vi "Example 3.vi"(8 "error in (no error)":errorcluster, 9 "export file path":path, 10 "target in":refnum<k24>, 11 "configuration file path":path) -> (0 "error out":errorcluster)   [LabVIEW 2018]
uses:
  NationalInstruments.VeriStand.SystemDefinitionAPI
  <vilib>/addons/VeriStand Custom Device Scripting APIs/Instrument Addon/API/TypeDefs/Message Settings.ctl
  <vilib>/addons/VeriStand Custom Device Scripting APIs/Instrument Addon/API/TypeDefs/Protection Types.ctl
  <vilib>/addons/VeriStand Custom Device Scripting APIs/Instrument Addon/API/TypeDefs/Single Channel Format Settings.ctl
  <vilib>/addons/VeriStand Custom Device Scripting APIs/Instrument Addon/API/TypeDefs/Command Settings.ctl
  <vilib>/NI Veristand/Custom Device API/Custom Device Item Ref.ctl
  <vilib>/addons/VeriStand Custom Device Scripting APIs/Instrument Addon/API/TypeDefs/Padding.ctl
  <vilib>/addons/VeriStand Custom Device Scripting APIs/Instrument Addon/API/TypeDefs/Array Type Cast Settings.ctl
  <vilib>/addons/VeriStand Custom Device Scripting APIs/Instrument Addon/API/TypeDefs/Array Element.ctl
  <vilib>/addons/VeriStand Custom Device Scripting APIs/Instrument Addon/Shared Directory/Type Cast Type.ctl
  <vilib>/addons/VeriStand Custom Device Scripting APIs/Instrument Addon/Shared Directory/Endian.ctl
  <vilib>/addons/VeriStand Custom Device Scripting APIs/Instrument Addon/API/Channels/Create Global MetaData Channel - Array - Type Cast.vi
  <vilib>/addons/VeriStand Custom Device Scripting APIs/Instrument Addon/API/Messages/Create Message - Value Change & Trigger.vi
  <vilib>/addons/VeriStand Custom Device Scripting APIs/Instrument Addon/API/Channels/Create MetaData Channel - Single Channel - Format.vi
  <vilib>/addons/VeriStand Custom Device Scripting APIs/Instrument Addon/API/Instrument Addon Scripting API.lvlib
  <vilib>/NI VeriStand/Custom Device API/Custom Device API.lvlib
  <vilib>/addons/VeriStand Custom Device Scripting APIs/Instrument Addon/Shared Directory/Instrument Addon Shared.lvlib
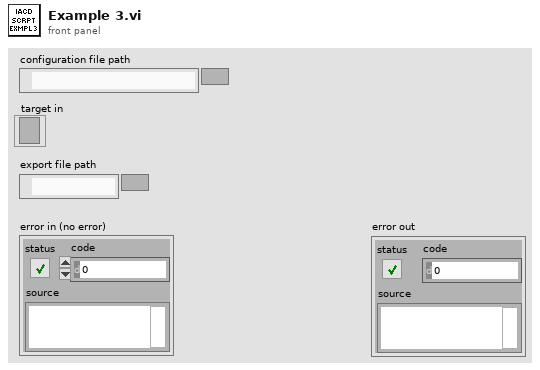
[diagram p1: front panel]
types:
  T1 = typedef "Custom Device API.lvlib/Custom Device Item Ref.ctl" = u64
  T2 = cluster{"Variable Name":string, "Channel Ref in":T1}
  T3 = typedef "Instrument Addon Scripting API.lvlib/Array Type Cast Settings.ctl" = cluster{"Elements":T4[], "Delimiter":string, "Type":T5, "Endian":T6}
  T4 = typedef "Instrument Addon Scripting API.lvlib/Array Element.ctl" = cluster{"Name":string, "Default Value":dbl, "Units":string}
  T5 = typedef "Instrument Addon Shared.lvlib/Type Cast Type.ctl" = enum16{"DBL", "SGL", "U64", "U32", "U16", "U8", "I64", "I32", "I16", "I8"}
  T6 = typedef "Instrument Addon Shared.lvlib/Endian.ctl" = enum16{"Native", "Little", "Big"}
  T7 = typedef "Instrument Addon Scripting API.lvlib/Padding.ctl" = cluster{"Pad Value":u8, "Length":u32}
  T8 = typedef "Instrument Addon Scripting API.lvlib/Command Settings.ctl" = cluster{"Command Format":string, "Linked Channels":cluster{"Variable Name":string, "Channel Ref in":T1}[], "Use Padding?":bool, "Padding":T7}
  T9 = typedef "Instrument Addon Scripting API.lvlib/Single Channel Format Settings.ctl" = cluster{"Format String":string, "Default Value":dbl, "Units":string}
  T10 = typedef "Instrument Addon Scripting API.lvlib/Message Settings.ctl" = cluster{"Protection":T11, "Enable Periodic Default":bool, "Trigger Channel refnum":u64}
  T11 = typedef "Instrument Addon Scripting API.lvlib/Protection Types.ctl" = enum16{"None", "CRC-32", "Checksum U16", "Checksum U32", "Checksum U8"}
  T12 = cluster{"Variable Name":string, "Channel Ref in":T1}[]
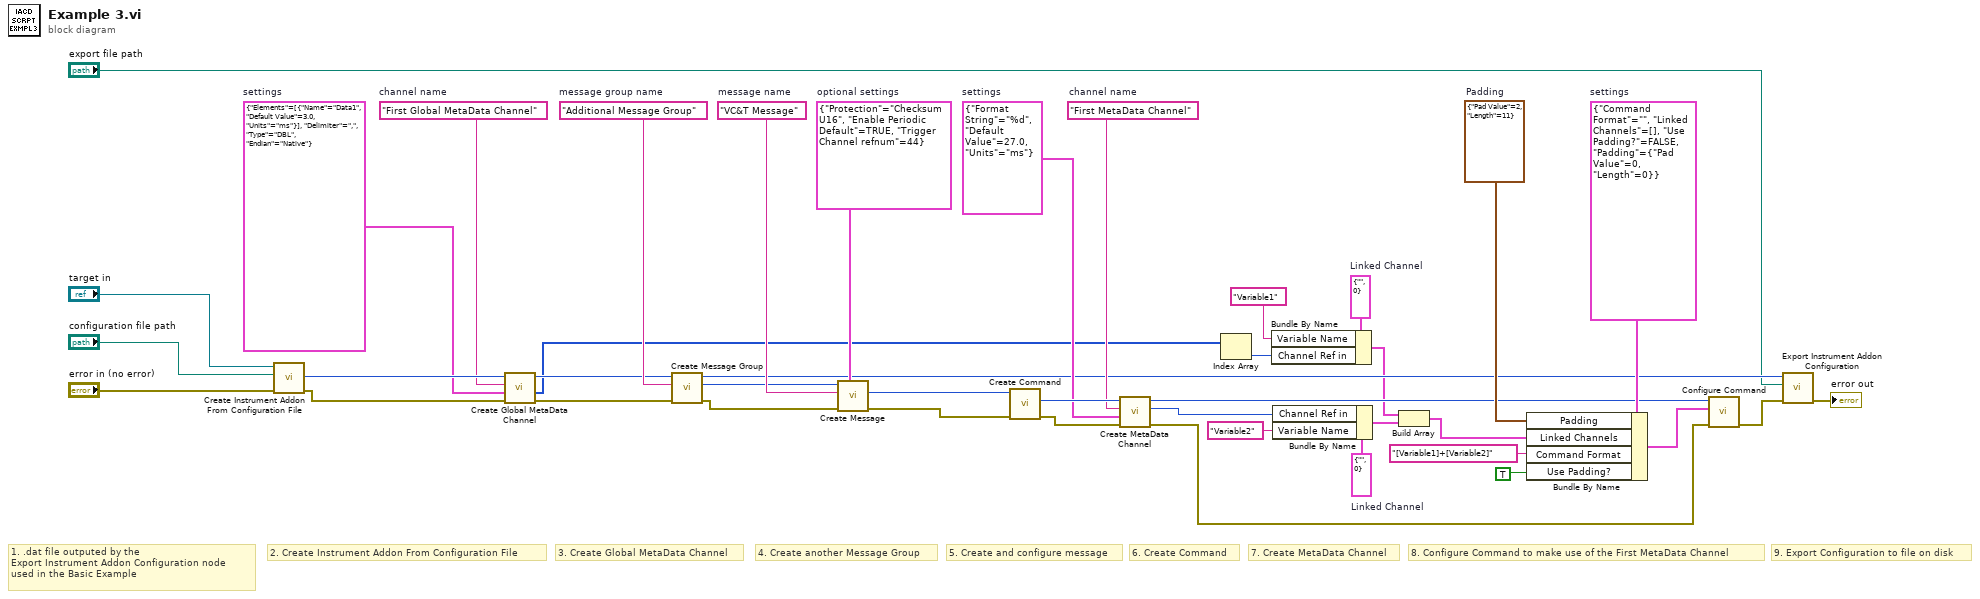
[diagram p0: block diagram]
diagram:
  w5 = T2 {"Variable Name"="", "Channel Ref in"=0}  # Linked Channel
  w7 = T3 {"Elements"=[{"Name"="Data1", "Default Value"=3.0, "Units"="ms"}], "Delimiter"=",", "Type"=enum."DBL", "Endian"=enum."Native"}  # settings
  w8 = "First Global MetaData Channel"  # channel name
  w21 = T7 {"Pad Value"=2, "Length"=11}  # Padding
  w27 = T2 {"Variable Name"="", "Channel Ref in"=0}  # Linked Channel
  w29 = T8 {"Command Format"="", "Linked Channels"=[], "Use Padding?"=FALSE, "Padding"={"Pad Value"=0, "Length"=0}}  # settings
  w31 = T9 {"Format String"="%d", "Default Value"=27.0, "Units"="ms"}  # settings
  w32 = "First MetaData Channel"  # channel name
  w35 = T10 {"Protection"=enum."Checksum U16", "Enable Periodic Default"=TRUE, "Trigger Channel refnum"=44}  # optional settings
  w37 = "VC&T Message"  # message name
  w38 = "Additional Message Group"  # message group name
  # "3. Create Global MetaData Channel"
  # "9. Export Configuration to file on disk"
  # "8. Configure Command to make use of the First MetaData Channel"
  # "7. Create MetaData Channel"
  # "6. Create Command"
  # "5. Create and configure message"
  # "4. Create another Message Group"
  # "2. Create Instrument Addon From Configuration File"
  # "1. .dat file outputed by the \nExport Instrument Addon Configuration node \nused in the Basic Example"
  n1 = call <vilib>:"Create Instrument Addon From Configuration File.vi"("error in (no error)"="error in (no error)", "configuration file path"="configuration file path", "target in"="target in") -> ("error out"=w10:errorcluster, "instrument addon refnum"=w12:T1)  [unwired: 6 in, 1 out]
  n2 = call-poly <vilib>:"Create Global MetaData Channel.vi"("error in (no error)"=w10, "settings"=w7, "channel name"=w8, "instrument addon refnum in"=w12) -> ("error out"=w9:errorcluster, "channel refnums"=w3:T1[], "instrument addon refnum out"=w11:T1)  [unwired: 4 in, 1 out]
  n3 = call <vilib>:"Create Message Group.vi"("error in (no error)"=w9, "message group name"=w38, "instrument addon refnum in"=w11) -> ("error out"=w34:errorcluster, "message group refnum out"=w36:T1, "instrument addon refnum out"=w15:T1)  [unwired: 6 in]
  n4 = call-poly <vilib>:"Create Message.vi"("optional settings"=w35, "error in (no error)"=w34, "message name"=w37, "message group refnum in"=w36) -> ("error out"=w20:errorcluster, "message refnum out"=w19:T1)  [unwired: 5 in, 1 out]
  n5 = call <vilib>:"Create Command.vi"("error in"=w20, "message refnum In"=w19) -> ("error out"=w30:errorcluster, "command refnum"=w33:T1)  [unwired: 7 in, 1 out]
  n6 = call-poly <vilib>:"Create MetaData Channel.vi"("error in (no error)"=w30, "settings"=w31, "channel name"=w32, "command refnum in"=w33) -> ("error out"=w16:errorcluster, "channel refnum"=w23:T1, "command refnum out"=w18:T1)  [unwired: 5 in]
  n7 = Index Array(array=w3) -> (element=w2:T1)  [unwired: 1 in]
  n8 = Bundle By Name(cluster=w5, "Variable Name"="Variable1", "Channel Ref in"=w2) -> (w1:T2)
  n9 = Bundle By Name(cluster=w27, "Channel Ref in"=w23, "Variable Name"="Variable2") -> (w25:T2)
  n10 = Build Array(w1, w25) -> (w24:T12)
  n11 = Bundle By Name(cluster=w29, "Padding"=w21, "Linked Channels"=w24, "Command Format"="[Variable1]+[Variable2]", "Use Padding?"=TRUE) -> (w17:T8)
  n12 = call <vilib>:"Configure Command.vi"("error in (no error)"=w16, "settings"=w17, "command refnum in"=w18) -> ("error out"=w14:errorcluster)  [unwired: 7 in, 1 out]
  n13 = call <vilib>:"Export Instrument Addon Configuration.vi"("error in (no error)"=w14, "export file path"="export file path", "instrument addon refnum in"=w15) -> ("error out"=→"error out":errorcluster)  [unwired: 7 in, 1 out]
